vi "FG.vi"() -> ()   [LabVIEW 2025]
uses:
  <vilib>/Instr/_visa.llb/VISA Configure Serial Port (Instr).vi
  <vilib>/measure/NI_MABase.lvlib
panel:
  in  "OK":bool
  out "Waveform Chart":waveform(dbl)(graph)
  in  "stop":bool
  out "wave":string
  in  "frequency":dbl
  in  "wave type":enum16{"triangle", "square", "sine"}(ring)
  in  "milliseconds to wait":u32
  in  "baud rate (9600)":u32=9600
  in  "VISA resource name":refnum<visa-resource-name>
  # "value"
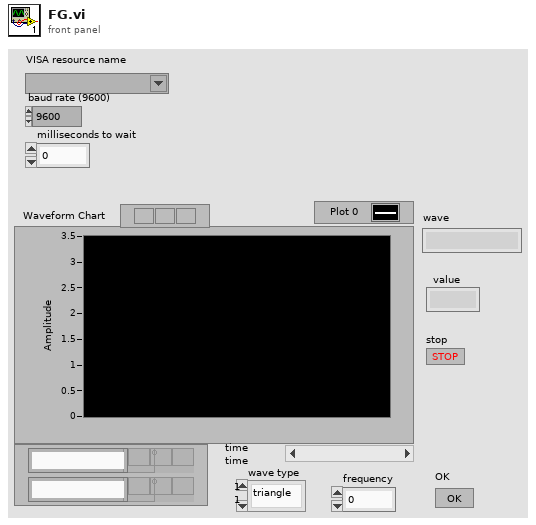
[diagram p1: front panel]
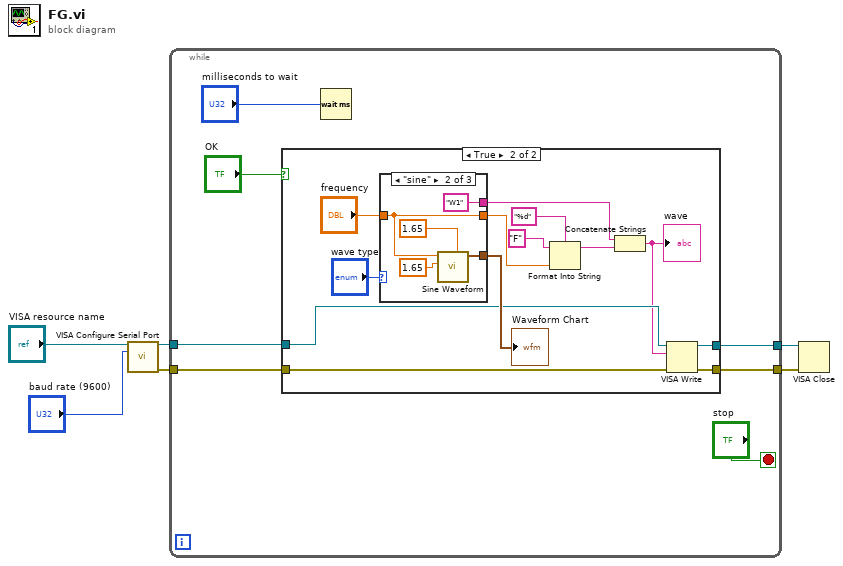
[diagram p0: block diagram]
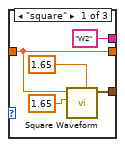
[diagram p3: hidden frame]
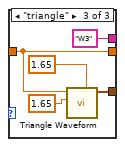
[diagram p4: hidden frame]
diagram:
  n1 = call-poly "VISA Configure Serial Port"("VISA resource name"="VISA resource name", "baud rate (9600)"="baud rate (9600)") -> ("VISA resource name out"=w4:refnum<visa-resource-name>, "error out"=w3:errorcluster)  [unwired: 12 in]
  n2 = while {
    tunnel: w4 -> [w11]
    tunnel: w3 -> [w10]
    tunnel: [w9] -> w2
    tunnel: [w8] -> w1
    stop <- "stop" stop-if-true
    n3 = case shown="True" "OK" {
      tunnel: w11 -> [w15 w20]
      tunnel: w10 -> [w14 w19]
      tunnel: [w15 w18] -> w9
      tunnel: [w14 w17] -> w8
      frame False {
      }
      frame True {
        n4 = case shown="\"sine\"" "wave type" {
          tunnel: ["W2" "W1" "W3"] -> w27
          tunnel: [w30 w36 w39] -> w26
          tunnel: [w29 w34 w40] -> w23
          tunnel: "frequency" -> [w29 w34 w40]
          frame "square" {
            n5 = call <vilib>:"Square Waveform.vi"("offset"=1.65 ("amplitude"), "amplitude"=1.65 ("offset"), "frequency"=w29) -> ("signal out"=w30:waveform(dbl))  [unwired: 7 in, 1 out]
          }
          frame "sine" {
            n6 = call <vilib>:"Sine Waveform.vi"("offset"=1.65, "amplitude"=1.65, "frequency"=w34) -> ("signal out"=w36:waveform(dbl))  [unwired: 7 in, 1 out]
          }
          frame "triangle" {
            n7 = call <vilib>:"Triangle Waveform.vi"("offset"=1.65 ("amplitude"), "amplitude"=1.65 ("offset"), "frequency"=w40) -> ("signal out"=w39:waveform(dbl))  [unwired: 7 in, 1 out]
          }
        }
        "Waveform Chart" <- w26
        n8 = Format Into String(format string="%d", initial string="F", w23) -> (resulting string=w22:string)  [unwired: 1 in, 1 out]
        n9 = Concatenate Strings(w27, w22) -> (w16:string)
        "wave" <- w16
        n10 = VISA Write(VISA resource name=w20, write buffer=w16, error in (no error)=w19) -> (VISA resource name out=w18:refnum<visa-resource-name>, error out=w17:errorcluster)  [unwired: 1 out]
      }
    }
    n11 = Wait (ms)(milliseconds to wait="milliseconds to wait") -> ()  [unwired: 1 out]
  }
  n12 = VISA Close(VISA resource name=w2, error in (no error)=w1) -> ()  [unwired: 1 out]
